vi "Display Result.vi"(0 "exponent":dbl, 11 "error in (no error)":errorcluster) -> (15 "error out":errorcluster)   [LabVIEW 2015]
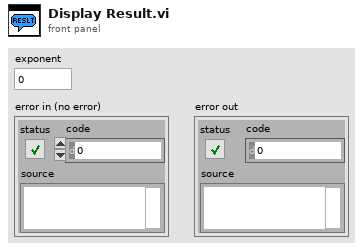
[diagram p1: front panel]
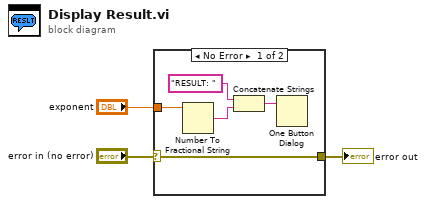
[diagram p0: block diagram]
diagram:
  n1 = case shown="No Error" "error in (no error)" {
    selector: "error in (no error)" -> [w7 w9]
    tunnel: "exponent" -> [w8 _]
    tunnel: [w7 w9] -> w1
    frame No Error {
      n2 = Number To Fractional String(number=w8) -> (F-format string=w6:string)  [unwired: 3 in]
      n3 = Concatenate Strings("RESULT: " ("string"), w6) -> (w5:string)
      n4 = One Button Dialog(message=w5) -> ()  [unwired: 1 in, 1 out]
    }
    frame Error {
    }
  }
  "error out" <- w1
